vi "VESASignal_CalcFramebufferAddress.vi"(1 "h_Pixel":i16, 4 "v_Pixel":i16) -> (14 "draw_pixel":bool, 15 "Address":u32, 16 "buffer":u8, 17 "h_sync":bool, 18 "v_sync":bool, 19 "Sub Buffer":u8)   [LabVIEW 2020]
uses:
  <vilib>/Utility/error.llb/Clear Errors.vi
  <vilib>/rvi/Emulation/niFpgaSctlEmulationGetInTimedLoop.vi
  <vilib>/rvi/Emulation/niFpgaEmulationIsFPGAContextNoSignature.vi
  <vilib>/rvi/DataTransferAndStorage/Container/Common/niFpgaContainerGetUniqueNameForEmu.vi
  <vilib>/rvi/Memory/Memory_Emulation/niFpgaMemoryEmulationCacheClearOnFirstRun.vi
  <vilib>/rvi/Memory/Memory_Emulation/nirvimemoryEmulationManagerCache_MakeExclusive.vi
  <vilib>/rvi/Memory/Memory_Emulation/niFpgaMemoryEmulationValidateCache.vi
  <vilib>/rvi/Memory/Memory_Emulation/nirvimemoryEmulationManagerCache_InsertValue.vi
  <vilib>/rvi/Memory/Memory_Emulation/nirvimemoryEmulationManagerCache_ReleaseExclusive.vi
  <vilib>/rvi/Memory/Memory_Emulation/nirvimemoryEmulationManagerCache_GetValue.vi
  <vilib>/rvi/Memory/Memory_Emulation/nirvimemoryEmulationManagerCache_SetValue.vi
  <vilib>/rvi/Emulation/niFpgaProcessEmulError.vi
  <vilib>/rvi/DataTransferAndStorage/Container/XNode/niFpgaContainer.xnode
  <vilib>/rvi/DataTransferAndStorage/Register/Emulation/niFpgaRegisterEmulation.vi
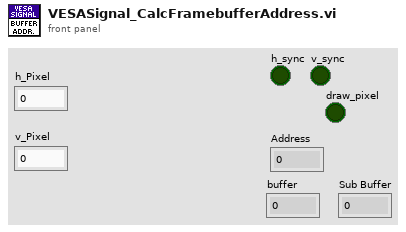
[diagram p1: front panel]
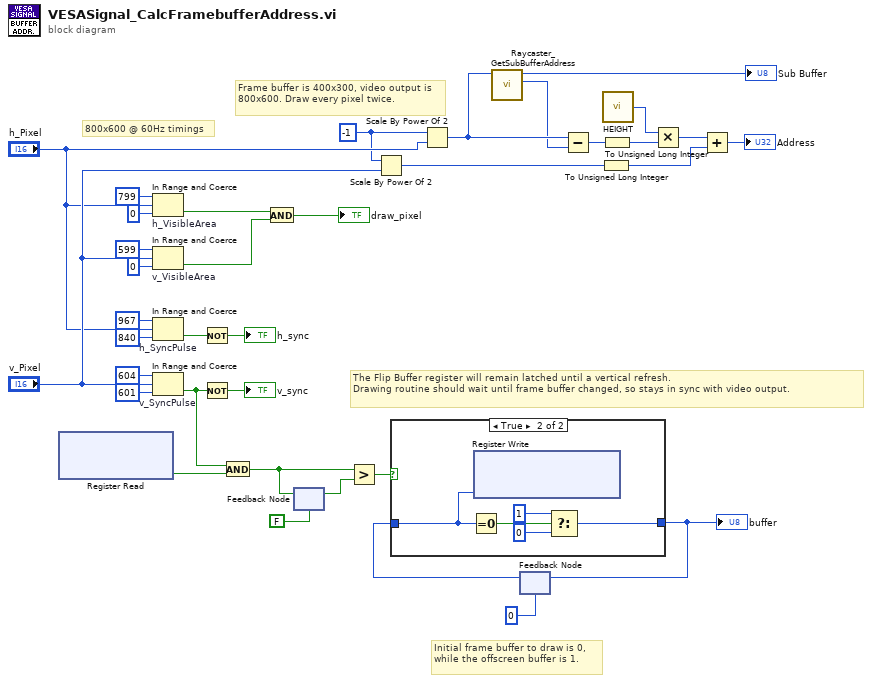
[diagram p0: block diagram]
diagram:
  w16 = i16 -1 ("n")
  # "800x600 @ 60Hz timings"
  # "Frame buffer is 400x300, video output is 800x600. Draw every pixel twice."
  # "Initial frame buffer to draw is 0, while the offscreen buffer is 1."
  # "The Flip Buffer register will remain latched until a vertical refresh.\nDrawing routine should wait until frame buffer changed, so stays in sync with video output."
  n1 = xnode "Register Read"() -> ("Data"=w11:bool)  [unwired: 1 in, 1 out]
  n2 = In Range and Coerce "h_VisibleArea"(upper limit=i16 799, x="h_Pixel", lower limit=i16 0) -> (In Range?=w27:bool)  [unwired: 1 out]
  n3 = In Range and Coerce "v_VisibleArea"(upper limit=i16 599, x="v_Pixel", lower limit=i16 0) -> (In Range?=w26:bool)  [unwired: 1 out]
  n4 = In Range and Coerce "h_SyncPulse"(upper limit=i16 967, x="h_Pixel", lower limit=i16 840) -> (In Range?=w34:bool)  [unwired: 1 out]
  n5 = In Range and Coerce "v_SyncPulse"(upper limit=i16 604, x="v_Pixel", lower limit=i16 601) -> (In Range?=w10:bool)  [unwired: 1 out]
  n6 = Not(x=w34) -> (.not. x?=→"h_sync":bool)
  n7 = Not(x=w10) -> (.not. x?=→"v_sync":bool)
  n8 = And(x=w10, y=w11) -> (x .and. y?=w9:bool)
  n9 = And(x=w27, y=w26) -> (x .and. y?=→"draw_pixel":bool)
  n10 = feedback #1(FALSE ("Data")) -> (w13:bool)
  n11 = feedback-in #1(w9) -> ()
  n12 = Greater?(x=w9, y=w13) -> (0:w12:bool)
  n13 = Scale By Power Of 2(n=w16, x="v_Pixel") -> (x*2^n=w17:i16)
  n14 = Scale By Power Of 2(n=w16, x="h_Pixel") -> (x*2^n=w3:i16)
  n15 = call "Raycaster_GetSubBufferAddress.vi"("Column"=w3) -> ("Start Address"=w2:i16, "Sub Buffer"=→"Sub Buffer":u8)  [unwired: 9 in]
  n16 = feedback #2(u8 0) -> (w23:u8)
  n17 = case shown="True" w12 {
    tunnel: w23 -> [w37 w42]
    tunnel: [w37 w38] -> w22
    frame False {
    }
    frame True {
      n18 = Equal To 0?(x=w42) -> (x = 0?=w41:bool)
      n19 = xnode ("Register Write")("Data"=w42) -> ()  [unwired: 1 in, 1 out]
      n20 = Select(t=u8 1, s=w41, f=u8 0) -> (s? t:f=w38:u8)
    }
  }
  "buffer" <- w22
  n21 = feedback-in #2(w22) -> ()
  n22 = Subtract(x=w3, y=w2) -> (x-y=w4:i16)
  n23 = To Unsigned Long Integer(number=w17) -> (unsigned 32bit integer=w5:u32)
  n24 = To Unsigned Long Integer(number=w4) -> (unsigned 32bit integer=w8:u32)
  n25 = call "HEIGHT.vi"() -> ("HEIGHT"=w7:i16)
  n26 = Multiply(x=w7, y=w8) -> (x*y=w6:u32)
  n27 = Add(x=w6, y=w5) -> (x+y=→"Address":u32)
